vi "Test Passing Pass If Equal Test.vi"(8 "error in (no error)":errorcluster, 11 "LUnit Test Case V2 Test Double In":refnum<class "Test Case Test Double.lvclass">) -> (0 "error out":errorcluster, 3 "LUnit Test Case V2 Test Double Out":refnum<class "Test Case Test Double.lvclass">)   [LabVIEW 2020, in "Test Case Test Double.lvclass"]
uses:
  Test Case Test Double.lvclass
  C:/Git/astemes-lunit/source/Rewrite Project/LUnit Test Case/LUnit Test Case V2.lvclass
  Core/LUnit Test Case/LUnit Test Case.lvclass/LUnit Test Case.ctl
  e088d5fe-0aa3-4de1-839d-1e2dad808fff.vi
  Core/LUnit Test Case/Private/Append Pass Result.vi
  Core/LUnit Test Case/Private/Append Fail Result.vi
  Core/LUnit Test Case/Private/Compare Variants.vi
  Core/LUnit Test Case/Private/Describe Comparison.vi
  Core/LUnit Test Case/Private/Variant to string.vi
  <vilib>/Utility/Data Type/Get Type Information.vi
  <vilib>/Utility/LVClass/Get LV Class Name.vi
  Test Case Test Double.lvclass/Test Case Test Double.ctl
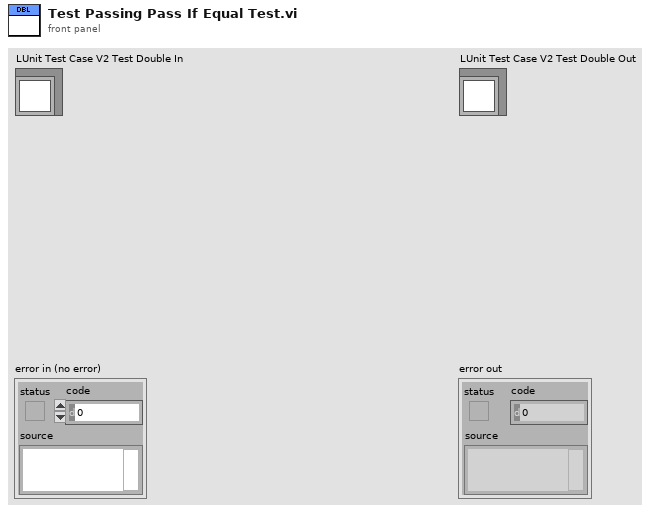
[diagram p1: front panel]
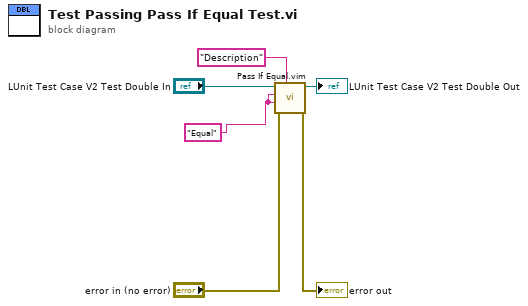
[diagram p0: block diagram]
diagram:
  w1 = "Equal"
  n1 = call "Pass If Equal.vim"("Description"="Description", "error in (no error)"="error in (no error)", "Actual"=w1, "Expected"=w1, "LUnit Test Case In"="LUnit Test Case V2 Test Double In") -> ("error out"=→"error out":errorcluster, "LUnit Test Case Out"=→"LUnit Test Case V2 Test Double Out":refnum<class "Test Case Test Double.lvclass">)  [unwired: 5 in]
